vi "set_power_track_on.vi"(8 "error in (no error)":errorcluster, 10 "POWER TRACK ON":bool, 11 "VISA resource name":refnum<visa-resource-name>) -> (0 "error out":errorcluster, 3 "VISA resource name out":refnum<visa-resource-name>)   [LabVIEW 2013]
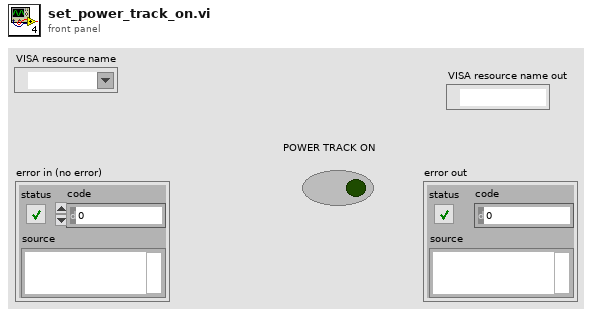
[diagram p1: front panel]
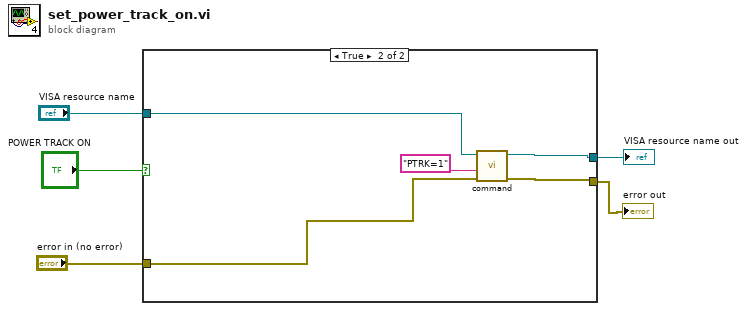
[diagram p0: block diagram]
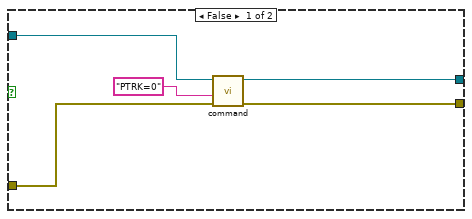
[diagram p2: hidden frame]
diagram:
  n1 = case shown="True" "POWER TRACK ON" {
    tunnel: "error in (no error)" -> [w9 w15]
    tunnel: "VISA resource name" -> [w10 w11]
    tunnel: [w7 w14] -> w2
    tunnel: [w6 w13] -> w1
    frame False {
      n2 = call "command.vi"("error in (no error)"=w9, "write buffer"="PTRK=0", "VISA resource name"=w10) -> ("error out"=w6:errorcluster, "VISA resource name out"=w7:refnum<visa-resource-name>)  [unwired: 7 in]
    }
    frame True {
      n3 = call "command.vi"("error in (no error)"=w15, "write buffer"="PTRK=1", "VISA resource name"=w11) -> ("error out"=w13:errorcluster, "VISA resource name out"=w14:refnum<visa-resource-name>)  [unwired: 7 in]
    }
  }
  "VISA resource name out" <- w2
  "error out" <- w1
